vi "SS Class Init.vi"(7 "VI Refnum":refnum<vi>, 8 "error in (no error)":errorcluster, 9 "Init Data":variant, 10 "Device":string, 11 "Subsystem CryoServer in":refnum<class "Subsystem CryoServer.lvclass">) -> (0 "error out":errorcluster, 2 "Channel List":refnum<class "HK Item.lvclass">[](array[class]), 3 "Subsystem CryoServer out":refnum<class "Subsystem CryoServer.lvclass">)   [LabVIEW 2021, in "Subsystem CryoServer.lvclass"]
uses:
  Subsystem CryoServer.lvclass
  hk-channel-class/HK Item/HK Item.lvclass
  Subsystem Class.lvclass
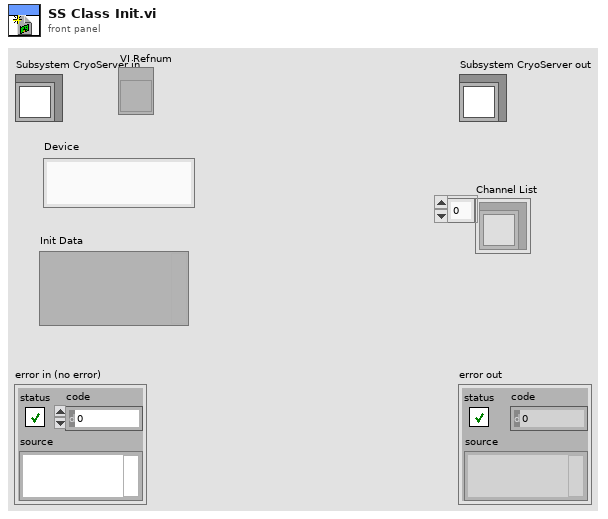
[diagram p1: front panel]
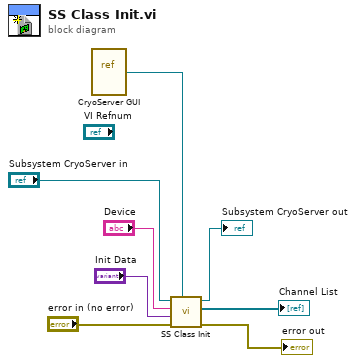
[diagram p0: block diagram]
diagram:
  n1 = vi-ref "CryoServer GUI.vi"() -> (w2:refnum<vi>)
  n2 = call-parent "SS Class Init.vi"("VI Refnum"=w2, "error in (no error)"="error in (no error)", "Init Data"="Init Data", "Device"="Device", "Subsystem Class in"="Subsystem CryoServer in") -> ("error out"=→"error out":errorcluster, "Channel List"=→"Channel List":refnum<class "HK Item.lvclass">[], "Subsystem Class out"=→"Subsystem CryoServer out":refnum<class "Subsystem CryoServer.lvclass">)  [unwired: 4 in]
